vi "2DPredictedClassification.vi"(8 "error in":errorcluster, 11 "Parameters":T1={"Plot"=refnum, "Data"={"X"=[], "Predict"=[]}, "Indexe"={"X"=0, "Y"=1}, "Point Property"={"Style"=enum."Full circle", "Label Color"=[8978528, 4367871, 1985280]}}) -> (0 "error out":errorcluster)   [LabVIEW 2020]
doc: "Displays predicted data based on trained data"
uses:
  Controls/PredictedParameter.ctl
  _Controls/Style.ctl
types:
  T1 = typedef "PredictedParameter.ctl" = cluster{"Plot":refnum<vi>, "Data":cluster{"X":dbl[][], "Predict":dbl[][]}, "Indexe":cluster{"X":i32, "Y":i32}, "Point Property":cluster{"Style":T2, "Label Color":u32[]}}
  T2 = typedef "Style.ctl" = enum16{"Empty circle", "Full circle", "Empty square", "Full square", "Cross"}
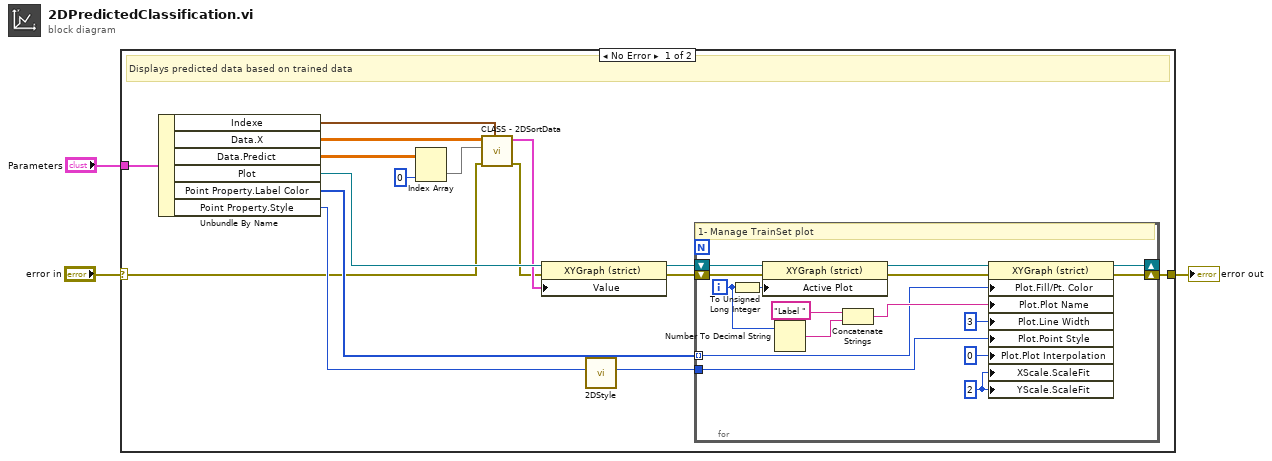
[diagram p0: block diagram]
diagram:
  n1 = case shown="No Error" "error in" {
    selector: "error in" -> [w5 w36]
    tunnel: "Parameters" -> [w18 _]
    tunnel: [w14 w36] -> w1
    frame No Error {
      # "Displays predicted data based on trained data"
      n2 = Unbundle By Name(w18) -> ("Indexe"=w6:cluster{"X":i32, "Y":i32}, "Data.X"=w11:dbl[][], "Data.Predict"=w10:dbl[][], "Plot"=w19:refnum<vi>, "Point Property.Label Color"=w15:u32[], "Point Property.Style"=w13:T2)
      n3 = Index Array(array=w10, index (col)=0 ("disabled index (col)")) -> (element=w8:dbl[])  [unwired: 1 in]
      n4 = call "CLASS - 2DSortData.vi"("Index"=w6, "error in"=w5, "Y"=w8, "X"=w11) -> ("error out"=w4:errorcluster, "Array"=w7:cluster{"Array":dbl[], "Array":dbl[]}[])  [unwired: 6 in]
      n5 = property class="XYGraph (strict)"(reference=w19, error in=w4, "Value"=w7) -> (reference out=w16:refnum<vi>, error out=w17:errorcluster)
      n6 = call "2DStyle.vi"("Style"=w13) -> ("Style"=w12:u8)  [unwired: 10 in]
      n7 = for {
        shift-right: [w25] -> w14
        shift-left: w17 -> [w34]
        shift-right: [w24] -> _
        shift-left: w16 -> [w35]
        tunnel: w12 -> [w21]
        tunnel: w15 -> [w20] mode=indexing
        i -> [w27]
        w23 = u8 2 ("X Scale.Scale Fit")
        # "1- Manage TrainSet plot"
        n8 = To Unsigned Long Integer(number=w27) -> (unsigned 32bit integer=w33:u32)
        n9 = property class="XYGraph (strict)"(reference=w35, error in=w34, "Active Plot"=w33) -> (reference out=w32:refnum<vi>, error out=w31:errorcluster)
        n10 = Number To Decimal String(number=w27) -> (decimal integer string=w29:string)  [unwired: 1 in]
        n11 = Concatenate Strings("Label " ("Plot.Plot Name"), w29) -> (w22:string)
        n12 = property class="XYGraph (strict)"(reference=w32, error in=w31, "Plot.Fill/Pt. Color"=w20, "Plot.Plot Name"=w22, "Plot.Line Width"=u8 3, "Plot.Point Style"=w21, "Plot.Plot Interpolation"=u8 0, "XScale.ScaleFit"=w23, "YScale.ScaleFit"=w23) -> (reference out=w24:refnum<vi>, error out=w25:errorcluster)
      }
    }
    frame Error {
    }
  }
  "error out" <- w1
